vi "Read ItemNames.vi"(8 "error in (no error)":errorcluster, 11 "BetterBoxHandle in":refnum<class "BetterBoxHandle.lvclass">) -> (0 "error out":errorcluster, 1 "Number of ItemNames":i32, 2 "Item Names":string[][](array[string]), 3 "BetterBoxHandle out":refnum<class "BetterBoxHandle.lvclass">)   [LabVIEW 2020, in "BetterDragAndDrop.lvlib" / "BetterBoxHandle.lvclass"]
uses:
  BetterBoxHandle.lvclass
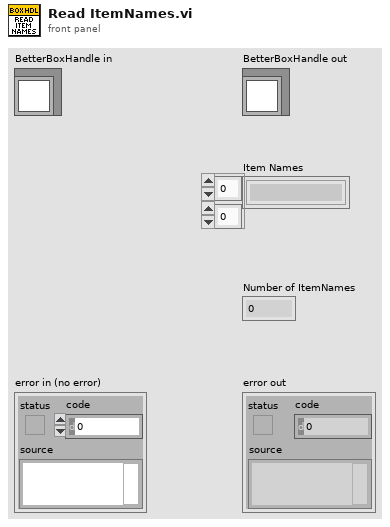
[diagram p1: front panel]
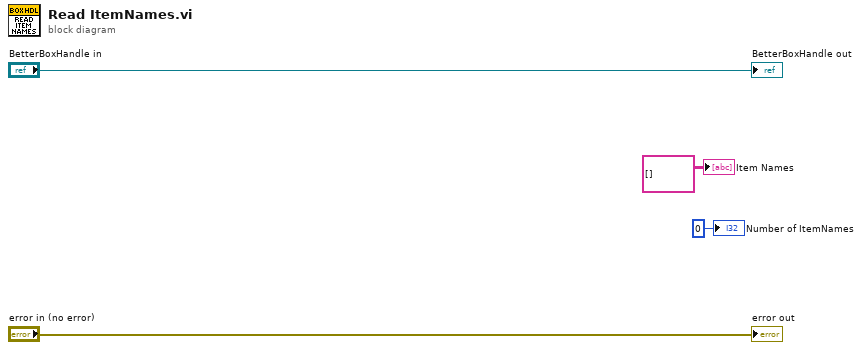
[diagram p0: block diagram]
diagram:
  "error out" <- "error in (no error)"
  "BetterBoxHandle out" <- "BetterBoxHandle in"
  "Item Names" <- string[][] [] ("Item Names")
  "Number of ItemNames" <- 0 ("Number of ItemNames")
